vi "Initialize.vi"(8 "error in (no error)":errorcluster, 11 "InsightCM Console Wrapper in":refnum<class "InsightCM Console Wrapper.lvclass">) -> (0 "error out":errorcluster, 3 "InsightCM Console Wrapper out":refnum<class "InsightCM Console Wrapper.lvclass">)   [LabVIEW 2020, in "InsightCM Console Wrapper.lvclass"]
doc: "Initializes the InsightCM Console Session. You need to call this VI before performing any other action with the console application."
uses:
  InsightCM Console Wrapper.lvclass
  C:/Users/fflores/Documents/GitHub Projects/LabVIEW-CLI-Wrapper/Console Wrapper/Console Wrapper.lvclass
  Console Wrapper/Console Wrapper.lvclass/Console Wrapper.ctl
  Console Wrapper/Write Application Name.vi
  Console Wrapper/Write Working Directory.vi
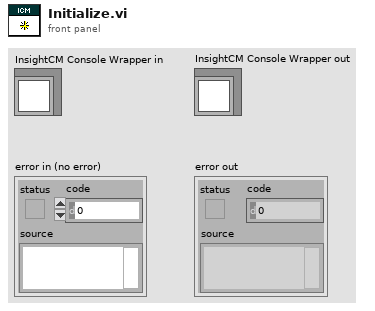
[diagram p1: front panel]
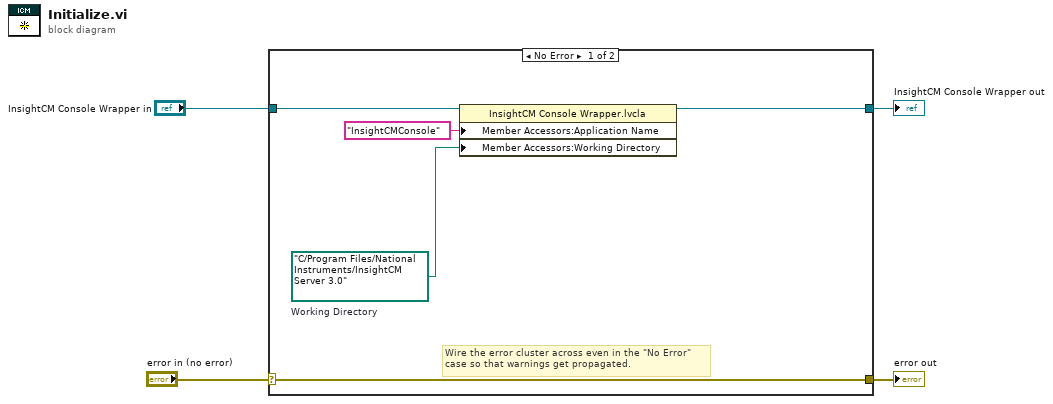
[diagram p0: block diagram]
diagram:
  n1 = case shown="No Error" "error in (no error)" {
    selector: "error in (no error)" -> [w8 w11]
    tunnel: [w8 w11] -> w3
    tunnel: [w7 w10] -> w1
    tunnel: "InsightCM Console Wrapper in" -> [w9 w10]
    frame No Error {
      w6 = path "C:/Program Files/National Instruments/InsightCM Server 3.0"  # Working Directory
      # "Wire the error cluster across even in the \"No Error\"\ncase so that warnings get propagated."
      n2 = property class="InsightCM Console Wrapper.lvcla"(reference=w9, "Member Accessors:Application Name"="InsightCMConsole" ("Application Name"), "Member Accessors:Working Directory"=w6) -> (reference out=w7:refnum<class "InsightCM Console Wrapper.lvclass">)  [unwired: 1 in, 1 out]
    }
    frame Error {
    }
  }
  "error out" <- w3
  "InsightCM Console Wrapper out" <- w1
